vi "Error handler.vi"(8 "error in (no error)":errorcluster, 9 "Clear errors":bool) -> (0 "error out":errorcluster, 3 "status":bool)   [LabVIEW 2014]
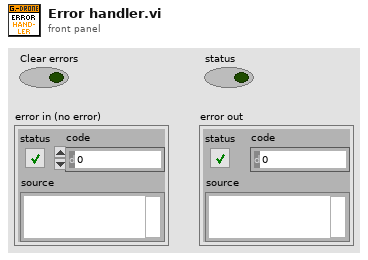
[diagram p1: front panel]
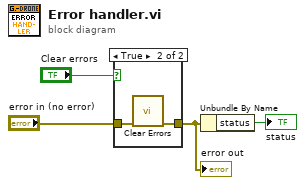
[diagram p0: block diagram]
diagram:
  n1 = case shown="True" "Clear errors" {
    tunnel: "error in (no error)" -> [w5 w7]
    tunnel: [w5 w6] -> w4
    frame False {
    }
    frame True {
      n2 = call <vilib>:"Clear Errors.vi"("error in (no error)"=w7) -> ("error out"=w6:errorcluster)  [unwired: 5 in, 1 out]
    }
  }
  "error out" <- w4
  n3 = Unbundle By Name(w4) -> ("status"=→"status":bool)
